vi "Flatten UIP Value.vi"(11 "Disabled UIP In":refnum<class "DisabledUIP.lvclass">) -> (0 "Error Out":errorcluster, 2 "String Value":string, 3 "Disabled UIP Out":refnum<class "DisabledUIP.lvclass">)   [LabVIEW 2015, in "DisabledUIP.lvclass"]
uses:
  DisabledUIP.lvclass
  DisabledUIP.lvclass/DisabledUIP.ctl
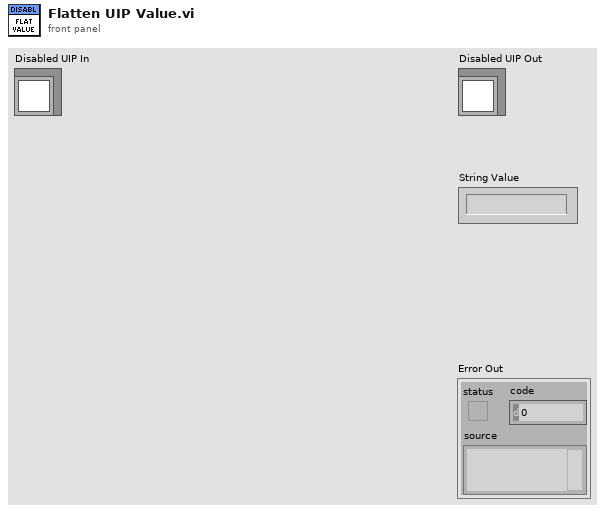
[diagram p1: front panel]
types:
  T1 = enum8{"Enabled", "Disabled", "Disabled and Grayed Out"}
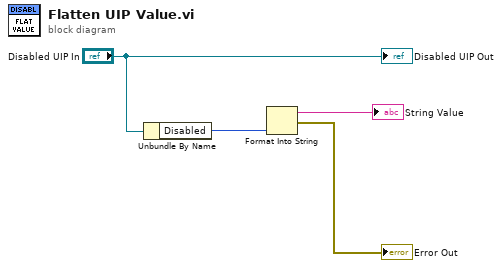
[diagram p0: block diagram]
diagram:
  n1 = Unbundle By Name("Disabled UIP In") -> ("Disabled"=w3:T1)
  n2 = Format Into String(w3) -> (resulting string=→"String Value":string, error out=→"Error Out":errorcluster)  [unwired: 3 in]
  "Disabled UIP Out" <- "Disabled UIP In"
